vi "transition.vi"(8 "error in (no error)":errorcluster, 10 "ContextData In":refnum<class "ContextData.lvclass">, 11 "Initialize in":refnum<class "Initialize.lvclass">) -> (0 "error out":errorcluster, 2 "ContextData Out":refnum<class "ContextData.lvclass">, 3 "Next State":refnum<class "State.lvclass">)   [LabVIEW 2018, in "Initialize.lvclass"]
uses:
  Initialize.lvclass
  ContextData/ContextData.lvclass
  State/State.lvclass
  Wait Event/Wait Event.lvclass
  C:/Users/fflores/Documents/OOP-State-Machine/State/State.lvclass
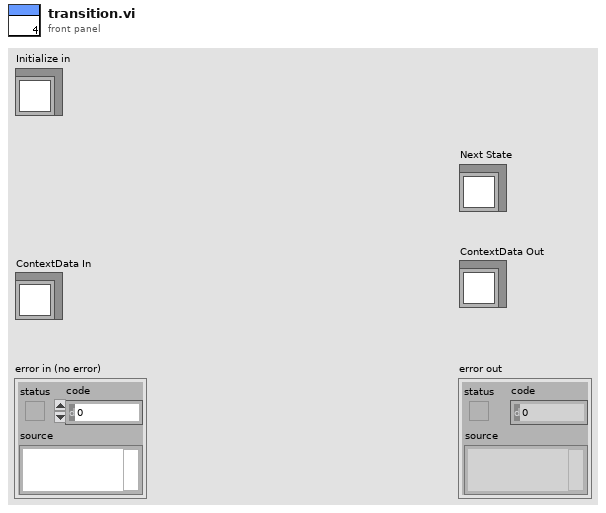
[diagram p1: front panel]
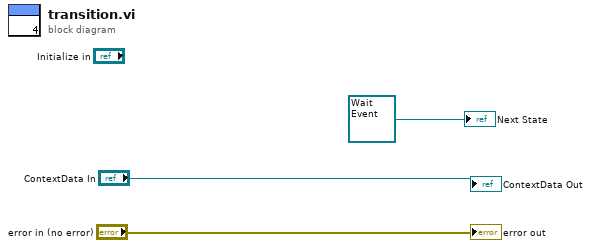
[diagram p0: block diagram]
diagram:
  "error out" <- "error in (no error)"
  "ContextData Out" <- "ContextData In"
  "Next State" <- refnum<class "Wait Event.lvclass"> refnum ("Wait Event.lvclass")
